vi "PID_controller_18.vi"() -> ()   [LabVIEW 2011]
panel:
  out "Angle (deg)":dbl format="%.1f"
  in  "Local":bool
  in  "Hold":bool
  out "tune_Method":u16(ring) items=["Setpoint", "Angle"]
  in  "Method":u16(ring)=1 items=["Setpoint", "Angle"]
  in  "Setpoint":u16(ring)=2 items=["A", "B", "C", "D"]
  out "do_tune":bool
  in  "Tune":bool
  out "Tune Set Point (torr)":dbl format="%.2f"
  in  "stop":bool
  out "fit":cluster{"element":dbl, "Value":dbl}[](array[cluster])
  out "err_avg":dbl
  out "Setpoint":string
  in  "Ks":dbl
  out "dt(s)":dbl
  out "windup error":dbl
  out "tPrev":dbl
  out "target value":dbl
  out "error(t-t0)":cluster{dbl, "Value":dbl}[](array[cluster])
  out "error":dbl
  out "tStart(s)":dbl
  out "S00":dbl
  out "S10":dbl
  out "S20":dbl
  out "S11":dbl
  out "S01":dbl
  out "weight":dbl[](array[numeric])
  in  "# of points to watch":i32=60
  in  "tSmooth(s)":dbl=4.0
  out "t0":dbl
  out "error(t)":cluster{dbl, "Value":dbl}[](array[cluster])
  out "IO error":errorcluster
  out "first":bool=TRUE
  out "XY Graph":T1(graph)
  out "current value":dbl
  in  "Period (s)":dbl=1.0
  out "dValue":dbl
  out "derivative":dbl
  out "integral":dbl
  in  "Angle (deg)":dbl format="%.1f"
  in  "Kd":dbl=0.4
  in  "Ki":dbl
  in  "Kp":dbl=0.1
  out "P (torr)":dbl format="%.2f"
  in  "Set Point (torr)":dbl format="%.2f"
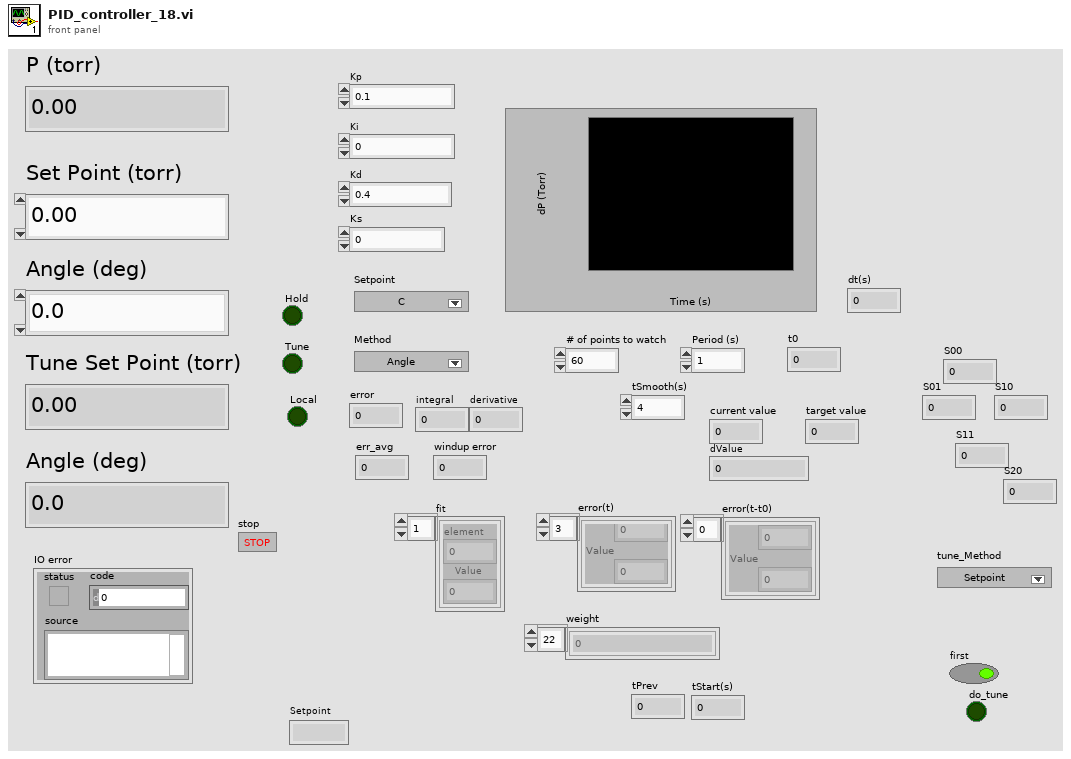
[diagram p1: front panel]
types:
  T1 = cluster{"Value":cluster{"element":dbl, "Value":dbl}[]}[]
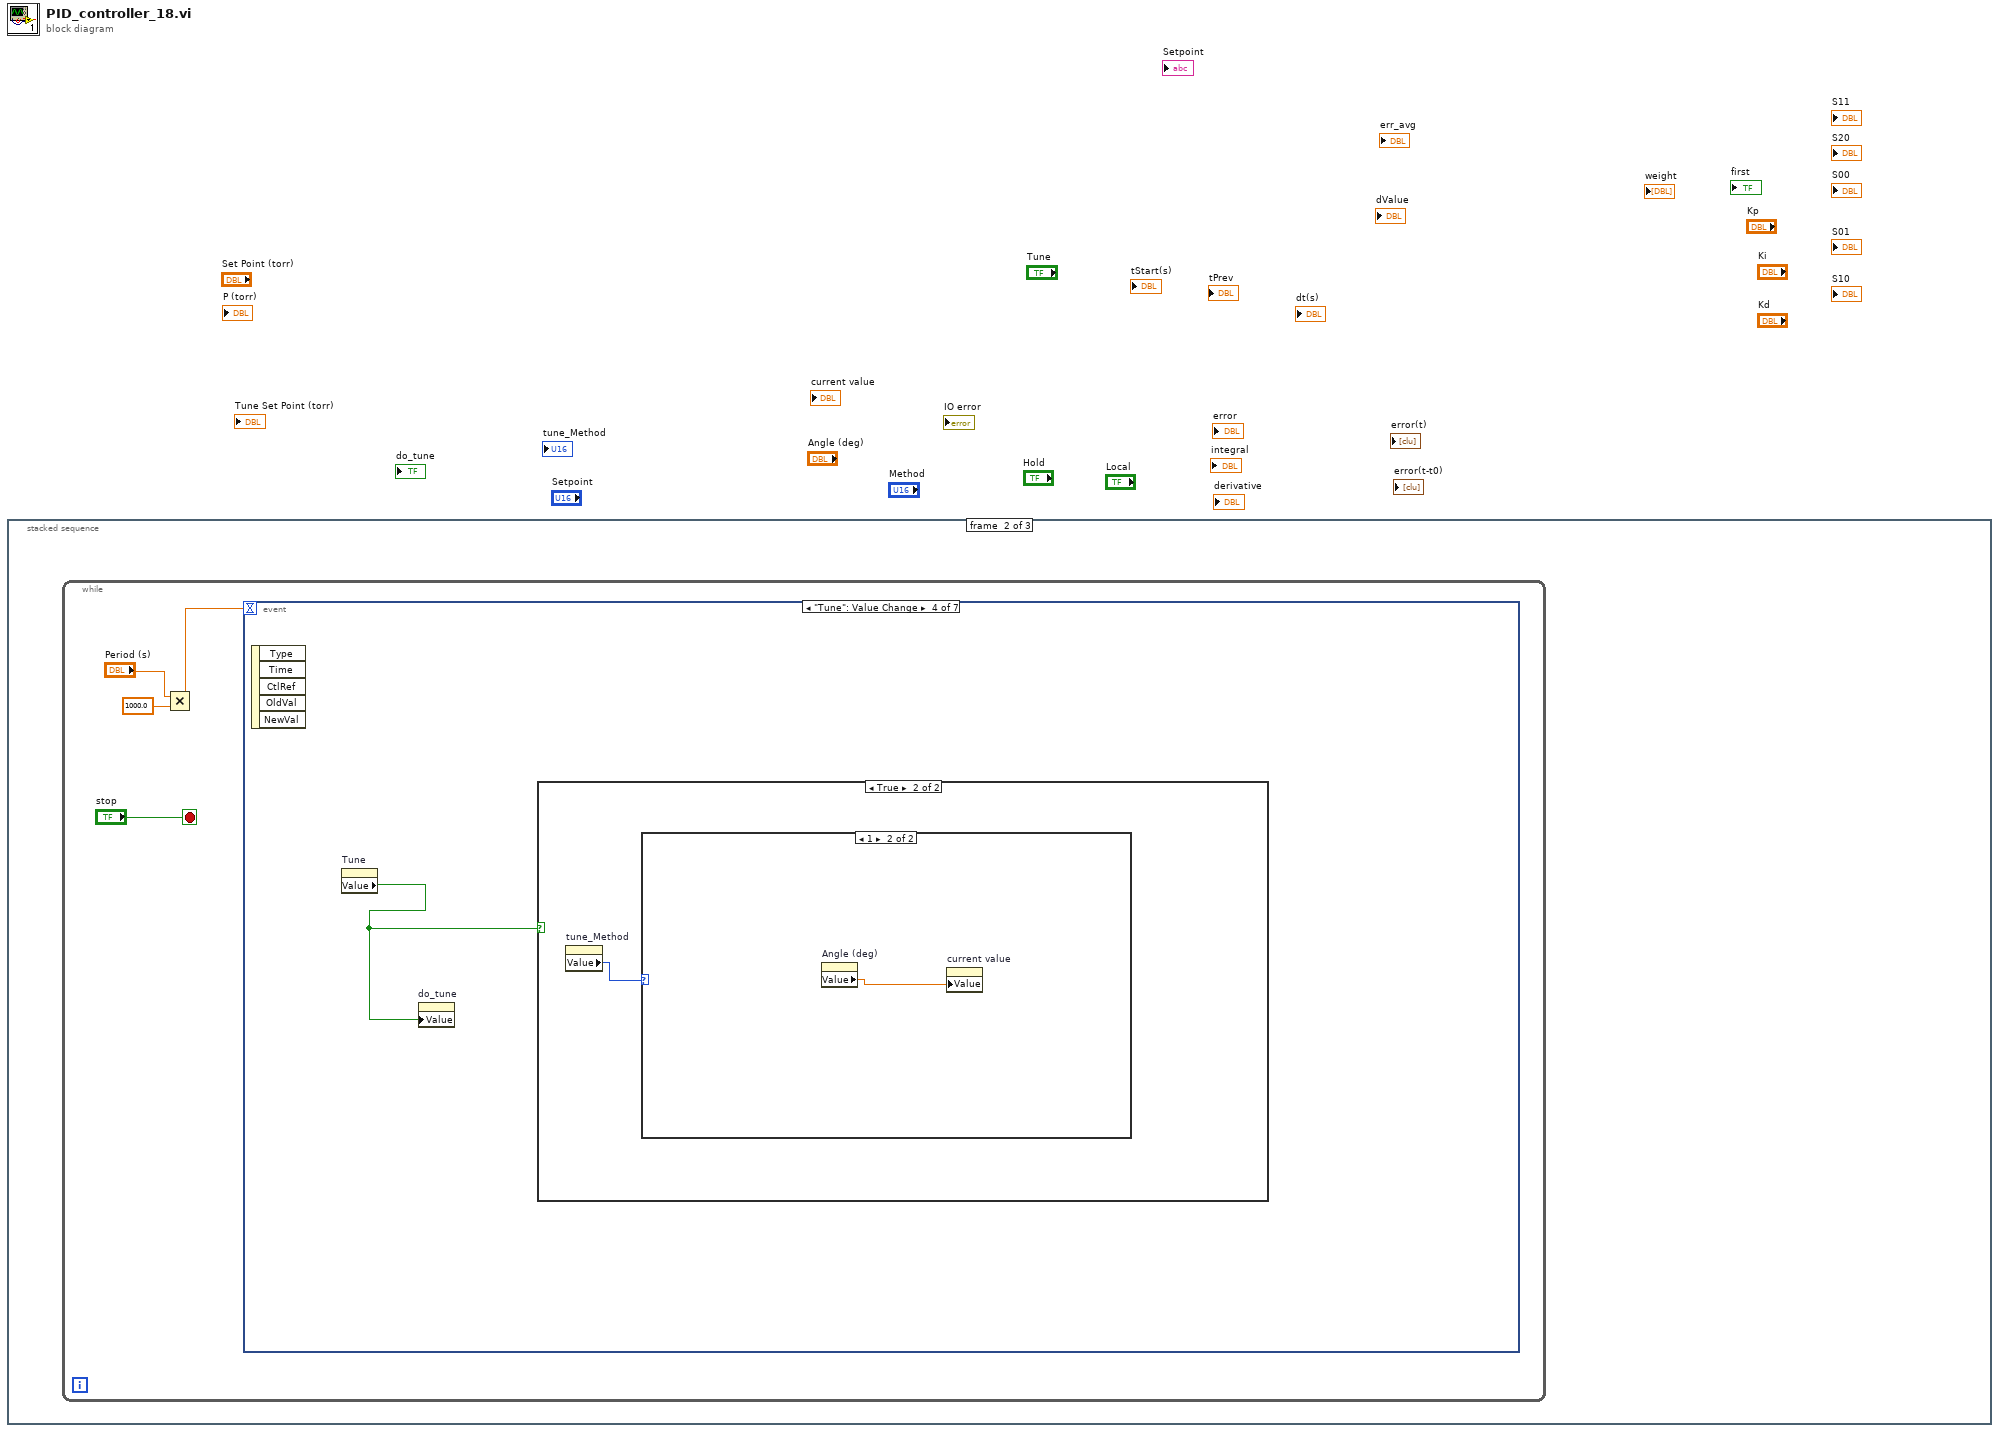
[diagram p0: block diagram]
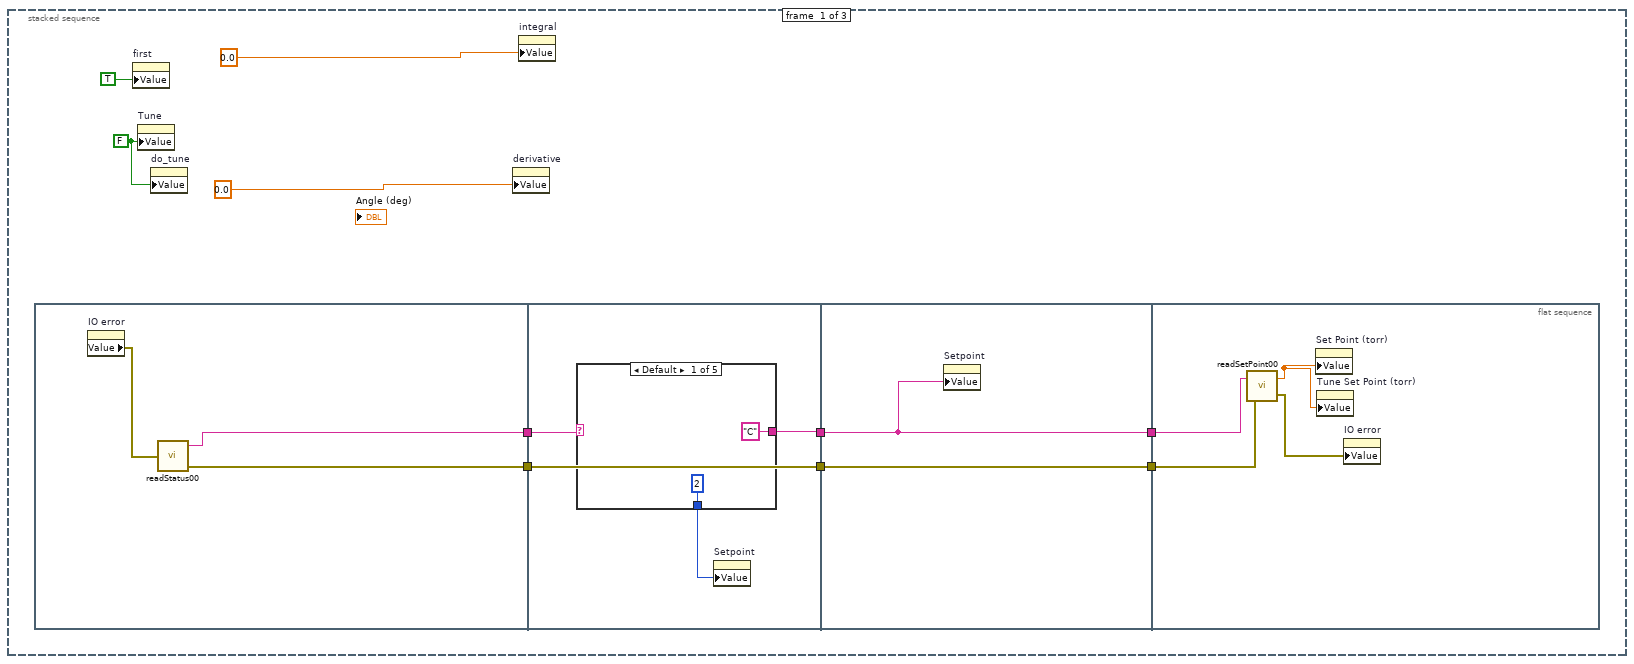
[diagram p2: hidden frame]
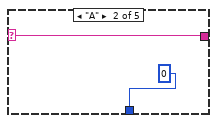
[diagram p3: hidden frame]
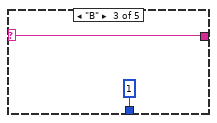
[diagram p4: hidden frame]
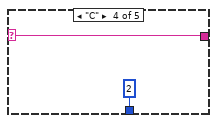
[diagram p5: hidden frame]
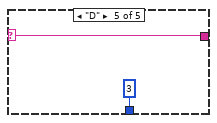
[diagram p6: hidden frame]
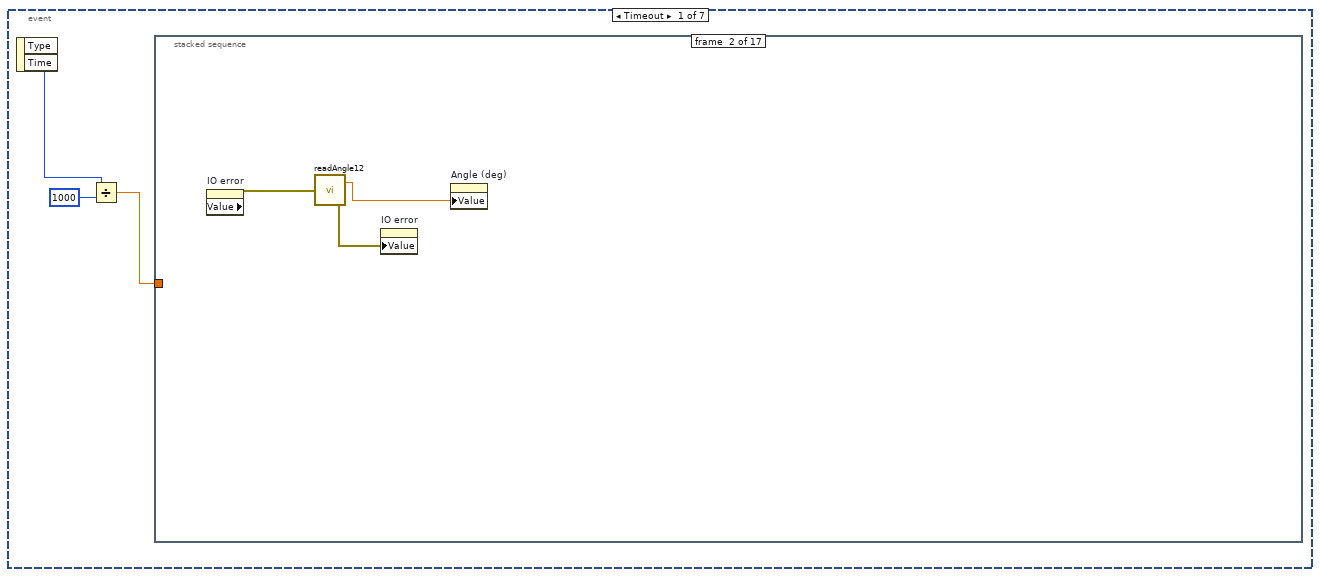
[diagram p7: hidden frame]
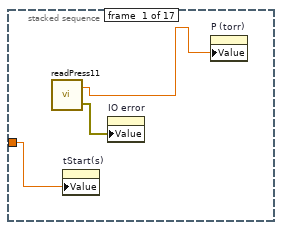
[diagram p8: hidden frame]
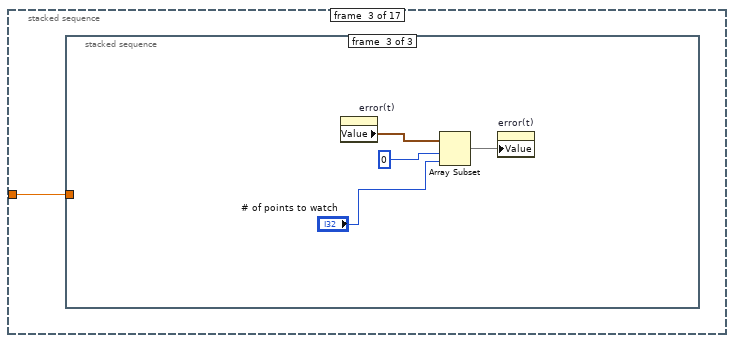
[diagram p9: hidden frame]
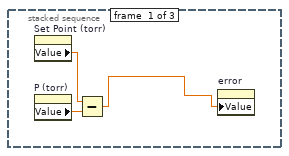
[diagram p10: hidden frame]
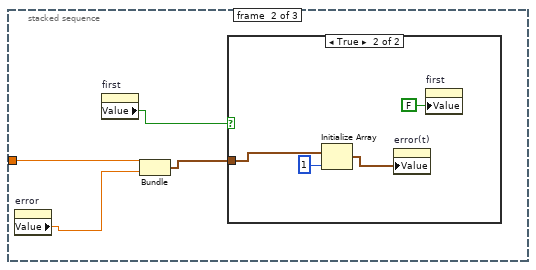
[diagram p11: hidden frame]
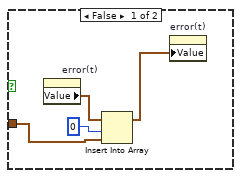
[diagram p12: hidden frame]
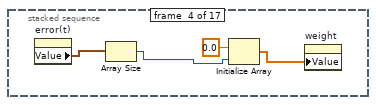
[diagram p13: hidden frame]
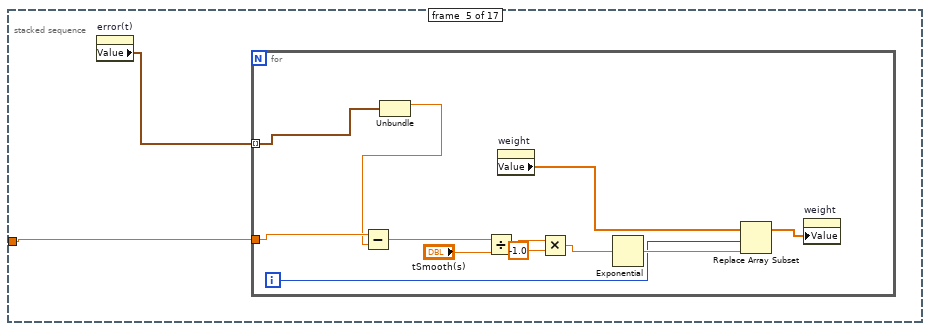
[diagram p14: hidden frame]
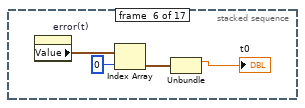
[diagram p15: hidden frame]
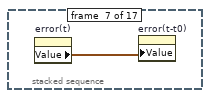
[diagram p16: hidden frame]
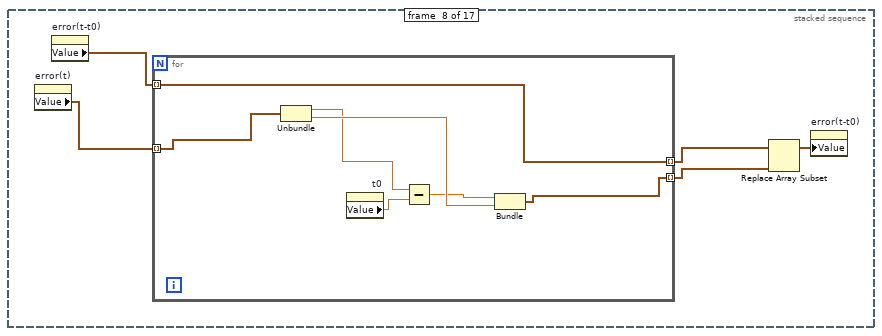
[diagram p17: hidden frame]
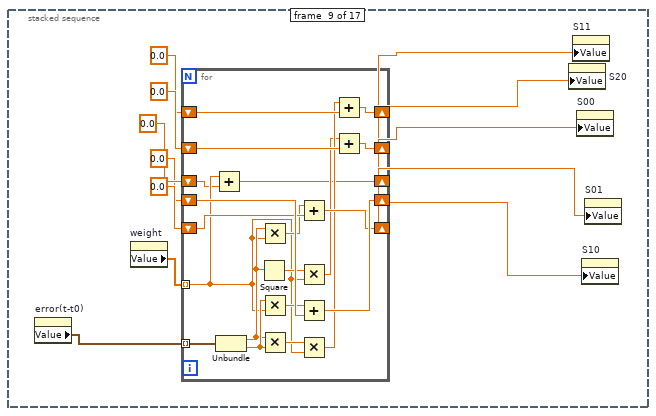
[diagram p18: hidden frame]
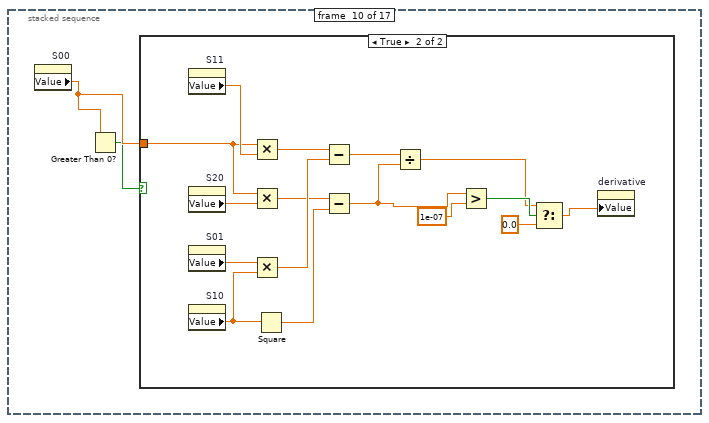
[diagram p19: hidden frame]
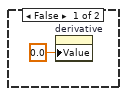
[diagram p20: hidden frame]
diagram:
  n1 = stacked-sequence {
    frame #0 {
      w7 = FALSE ("Tune")
      n2 = flat-sequence {
        tunnel: [w12] -> w6
        tunnel: [w11] -> w5
        tunnel: w6 -> [w16]
        tunnel: [w15] -> w4
        tunnel: w5 -> [w17]
        tunnel: [w17] -> w2
        tunnel: w4 -> [w28]
        tunnel: [w28] -> w3
        tunnel: w2 -> [w29]
        tunnel: [w29] -> w1
        tunnel: w3 -> [w33]
        tunnel: w1 -> [w32]
        frame #0 {
          n3 = property on="IO error" class="Clust (strict)"() -> ("Value"=w13:errorcluster)  [unwired: 2 in, 2 out]
          n4 = call "readStatus00.vi"("error in"=w13) -> ("Setpoint"=w12:string, "error out"=w11:errorcluster)  [unwired: 1 out]
        }
        frame #1 {
          n5 = case shown="Default" w16 {
            selector: w16 -> [_ w21 w22 w24 w26]
            tunnel: ["C" w21 w22 w24 w26] -> w15
            tunnel: [u16 2 ("Ring") u16 0 ("Ring") u16 1 ("Ring") u16 2 ("Ring") u16 3 ("Ring")] -> w14
            frame Default {
            }
            frame "A" {
            }
            frame "B" {
            }
            frame "C" {
            }
            frame "D" {
            }
          }
          n6 = property on="Setpoint" class="Ring (strict)"("Value"=w14) -> ()  [unwired: 2 in, 2 out]
        }
        frame #2 {
          n7 = property on="Setpoint" class="Str"("Value"=w28) -> ()  [unwired: 2 in, 2 out]
        }
        frame #3 {
          n8 = call "readSetPoint00.vi"("error in"=w32, "Setpoint"=w33) -> ("error out"=w31:errorcluster, "P"=w30:dbl)
          n9 = property on="Set Point (torr)" class="DigNum (strict)"("Value"=w30) -> ()  [unwired: 2 in, 2 out]
          n10 = property on="Tune Set Point (torr)" class="DigNum (strict)"("Value"=w30) -> ()  [unwired: 2 in, 2 out]
          n11 = property on="IO error" class="Clust (strict)"("Value"=w31) -> ()  [unwired: 2 in, 2 out]
        }
      }
      n12 = property on="first" class="Bool (strict)"("Value"=TRUE ("first")) -> ()  [unwired: 2 in, 2 out]
      n13 = property on="Tune" class="Bool (strict)"("Value"=w7) -> ()  [unwired: 2 in, 2 out]
      n14 = property on="do_tune" class="Bool (strict)"("Value"=w7) -> ()  [unwired: 2 in, 2 out]
      n15 = property on="derivative" class="DigNum (strict)"("Value"=0.0 ("derivative")) -> ()  [unwired: 2 in, 2 out]
      n16 = property on="integral" class="DigNum (strict)"("Value"=0.0 ("integral")) -> ()  [unwired: 2 in, 2 out]
    }
    frame #1 {
      n17 = while {
        stop <- "stop" stop-if-true
        n18 = Multiply(x="Period (s)", y=1000.0) -> (x*y=w35:dbl)
        n19 = event shown="[3] \"Tune\": Value Change" {
          selector: _ -> [_ _ _ _ _ _ _]
          dyn-events: _ -> [_ _ _ _ _ _ _]
          timeout: w35 -> [_ _ _ _ _ _ _]
          event Timeout {
            n20 = event-data() -> ("Time"=w40:u32)  [unwired: 1 in, 1 out]
            n21 = Divide(x=w40, y=u32 1000) -> (x/y=w38:dbl)
            n22 = stacked-sequence {
              tunnel: w38 -> [w41 _ w47 _ w71 _ _ _ _ _ _ _ _ _ _ _ _]
              frame #0 {
                n23 = call "readPress11.vi"() -> ("P"=w43:dbl, "error out"=w42:errorcluster)  [unwired: 1 in]
                n24 = property on="tStart(s)" class="DigNum (strict)"("Value"=w41) -> ()  [unwired: 2 in, 2 out]
                n25 = property on="IO error" class="Clust (strict)"("Value"=w42) -> ()  [unwired: 2 in, 2 out]
                n26 = property on="P (torr)" class="DigNum (strict)"("Value"=w43) -> ()  [unwired: 2 in, 2 out]
              }
              frame #1 {
                n27 = property on="IO error" class="Clust (strict)"() -> ("Value"=w45:errorcluster)  [unwired: 2 in, 2 out]
                n28 = call "readAngle12.vi"("error in"=w45) -> ("angle"=w46:dbl, "error out"=w44:errorcluster)
                n29 = property on="IO error" class="Clust (strict)"("Value"=w44) -> ()  [unwired: 2 in, 2 out]
                n30 = property on="Angle (deg)" class="DigNum (strict)"("Value"=w46) -> ()  [unwired: 2 in, 2 out]
              }
              frame #2 {
                n31 = stacked-sequence {
                  tunnel: w47 -> [_ w53 _]
                  frame #0 {
                    n32 = property on="Set Point (torr)" class="DigNum (strict)"() -> ("Value"=w49:dbl)  [unwired: 2 in, 2 out]
                    n33 = property on="P (torr)" class="DigNum (strict)"() -> ("Value"=w50:dbl)  [unwired: 2 in, 2 out]
                    n34 = Subtract(x=w49, y=w50) -> (x-y=w48:dbl)
                    n35 = property on="error" class="DigNum (strict)"("Value"=w48) -> ()  [unwired: 2 in, 2 out]
                  }
                  frame #1 {
                    n36 = property on="error" class="DigNum (strict)"() -> ("Value"=w51:dbl)  [unwired: 2 in, 2 out]
                    n37 = property on="first" class="Bool (strict)"() -> ("Value"=w54:bool)  [unwired: 2 in, 2 out]
                    n38 = Bundle(w53, "Value"=w51) -> (w52:cluster{dbl, "Value":dbl})  [unwired: 1 in]
                    n39 = case shown="True" w54 {
                      tunnel: w52 -> [w56 w61]
                      frame False {
                        n40 = property on="error(t)" class="Arr (strict)"() -> ("Value"=w57:cluster{dbl, "Value":dbl}[])  [unwired: 2 in, 2 out]
                        n41 = Insert Into Array(array=w57, index=0, new element=w56) -> (w55:cluster{dbl, "Value":dbl}[])
                        n42 = property on="error(t)" class="Arr (strict)"("Value"=w55) -> ()  [unwired: 2 in, 2 out]
                      }
                      frame True {
                        n43 = Initialize Array(w61, 1 ("dimension size")) -> (w59:cluster{dbl, "Value":dbl}[])
                        n44 = property on="error(t)" class="Arr (strict)"("Value"=w59) -> ()  [unwired: 2 in, 2 out]
                        n45 = property on="first" class="Bool (strict)"("Value"=FALSE ("first")) -> ()  [unwired: 2 in, 2 out]
                      }
                    }
                  }
                  frame #2 {
                    n46 = property on="error(t)" class="Arr (strict)"() -> ("Value"=w64:cluster{dbl, "Value":dbl}[])  [unwired: 2 in, 2 out]
                    n47 = Array Subset(array=w64, index=0, length="# of points to watch") -> (w66:cluster{dbl, "Value":dbl}[])
                    n48 = property on="error(t)" class="Arr (strict)"("Value"=w66) -> ()  [unwired: 2 in, 2 out]
                  }
                }
              }
              frame #3 {
                n49 = property on="error(t)" class="Arr (strict)"() -> ("Value"=w67:cluster{dbl, "Value":dbl}[])  [unwired: 2 in, 2 out]
                n50 = Array Size(array=w67) -> (size(s)=w69:i32)
                n51 = Initialize Array(0.0 ("element"), w69) -> (w70:dbl[])
                n52 = property on="weight" class="Arr (strict)"("Value"=w70) -> ()  [unwired: 2 in, 2 out]
              }
              frame #4 {
                n53 = property on="error(t)" class="Arr (strict)"() -> ("Value"=w72:cluster{dbl, "Value":dbl}[])  [unwired: 2 in, 2 out]
                n54 = for {
                  tunnel: w72 -> [w84] mode=indexing
                  tunnel: w71 -> [w83]
                  i -> [w79]
                  n55 = Unbundle(w84) -> (w82:dbl)  [unwired: 1 out]
                  n56 = Subtract(x=w83, y=w82) -> (x-y=w77:dbl)
                  n57 = Divide(x=w77, y="tSmooth(s)") -> (x/y=w75:dbl)
                  n58 = property on="weight" class="Arr (strict)"() -> ("Value"=w80:dbl[])  [unwired: 2 in, 2 out]
                  n59 = Multiply(x=w75, y=-1.0) -> (x*y=w73:dbl)
                  n60 = Exponential(1:w73) -> (0:w81:dbl)
                  n61 = Replace Array Subset(array=w80, new element=w81, index=w79) -> (w78:dbl[])
                  n62 = property on="weight" class="Arr (strict)"("Value"=w78) -> ()  [unwired: 2 in, 2 out]
                }
              }
              frame #5 {
                n63 = property on="error(t)" class="Arr (strict)"() -> ("Value"=w85:cluster{dbl, "Value":dbl}[])  [unwired: 2 in, 2 out]
                n64 = Index Array(array=w85, index=0) -> (element=w87:cluster{dbl, "Value":dbl})
                n65 = Unbundle(w87) -> (→"t0":dbl)  [unwired: 1 out]
              }
              frame #6 {
                n66 = property on="error(t)" class="Arr (strict)"() -> ("Value"=w89:cluster{dbl, "Value":dbl}[])  [unwired: 2 in, 2 out]
                n67 = property on="error(t-t0)" class="Arr (strict)"("Value"=w89) -> ()  [unwired: 2 in, 2 out]
              }
              frame #7 {
                n68 = property on="error(t)" class="Arr (strict)"() -> ("Value"=w90:cluster{dbl, "Value":dbl}[])  [unwired: 2 in, 2 out]
                n69 = property on="error(t-t0)" class="Arr (strict)"() -> ("Value"=w92:cluster{dbl, "Value":dbl}[])  [unwired: 2 in, 2 out]
                n70 = for {
                  tunnel: w90 -> [w97] mode=indexing
                  tunnel: [w96] -> w91 mode=indexing
                  tunnel: w92 -> [w95] mode=indexing
                  tunnel: [w95] -> w93 mode=indexing
                  n71 = Unbundle(w97) -> (w98:dbl, "Value"=w100:dbl)
                  n72 = property on="t0" class="DigNum (strict)"() -> ("Value"=w101:dbl)  [unwired: 2 in, 2 out]
                  n73 = Subtract(x=w98, y=w101) -> (x-y=w99:dbl)
                  n74 = Bundle(w99, "Value"=w100) -> (w96:cluster{dbl, "Value":dbl})  [unwired: 1 in]
                }
                n75 = Replace Array Subset(array=w93, new element=w91) -> (w94:cluster{dbl, "Value":dbl}[])  [unwired: 1 in]
                n76 = property on="error(t-t0)" class="Arr (strict)"("Value"=w94) -> ()  [unwired: 2 in, 2 out]
              }
              frame #8 {
                n77 = property on="error(t-t0)" class="Arr (strict)"() -> ("Value"=w113:cluster{dbl, "Value":dbl}[])  [unwired: 2 in, 2 out]
                n78 = property on="weight" class="Arr (strict)"() -> ("Value"=w106:dbl[])  [unwired: 2 in, 2 out]
                n79 = for {
                  tunnel: w113 -> [w129] mode=indexing
                  shift-right: [w130] -> w111
                  shift-left: 0.0 -> [w133]
                  shift-right: [w126] -> w108
                  shift-left: 0.0 -> [w132]
                  shift-right: [w125] -> w109
                  shift-left: 0.0 -> [w131]
                  shift-right: [w127] -> w112
                  shift-left: 0.0 -> [w128]
                  tunnel: w106 -> [w116] mode=indexing
                  shift-right: [w114] -> w110
                  shift-left: 0.0 -> [w115]
                  n80 = Add(x=w116, y=w115) -> (x+y=w114:dbl)
                  n81 = Unbundle(w129) -> (w118:dbl, "Value"=w124:dbl)
                  n82 = Square(x=w118) -> (x^2=w120:dbl)
                  n83 = Multiply(x=w118, y=w116) -> (x*y=w117:dbl)
                  n84 = Multiply(x=w124, y=w116) -> (x*y=w123:dbl)
                  n85 = Multiply(x=w118, y=w124) -> (x*y=w122:dbl)
                  n86 = Add(x=w117, y=w128) -> (x+y=w127:dbl)
                  n87 = Multiply(x=w120, y=w116) -> (x*y=w119:dbl)
                  n88 = Add(x=w123, y=w133) -> (x+y=w130:dbl)
                  n89 = Multiply(x=w122, y=w116) -> (x*y=w121:dbl)
                  n90 = Add(x=w121, y=w132) -> (x+y=w126:dbl)
                  n91 = Add(x=w119, y=w131) -> (x+y=w125:dbl)
                }
                n92 = property on="S20" class="DigNum (strict)"("Value"=w109) -> ()  [unwired: 2 in, 2 out]
                n93 = property on="S11" class="DigNum (strict)"("Value"=w108) -> ()  [unwired: 2 in, 2 out]
                n94 = property on="S00" class="DigNum (strict)"("Value"=w110) -> ()  [unwired: 2 in, 2 out]
                n95 = property on="S10" class="DigNum (strict)"("Value"=w112) -> ()  [unwired: 2 in, 2 out]
                n96 = property on="S01" class="DigNum (strict)"("Value"=w111) -> ()  [unwired: 2 in, 2 out]
              }
              frame #9 {
                n97 = property on="S00" class="DigNum (strict)"() -> ("Value"=w135:dbl)  [unwired: 2 in, 2 out]
                n98 = Greater Than 0?(x=w135) -> (x > 0?=w134:bool)
                n99 = case shown="True" w134 {
                  tunnel: w135 -> [_ w144]
                  frame False {
                    n100 = property on="derivative" class="DigNum (strict)"("Value"=0.0 ("derivative")) -> ()  [unwired: 2 in, 2 out]
                  }
                  frame True {
                    n101 = property on="S11" class="DigNum (strict)"() -> ("Value"=w146:dbl)  [unwired: 2 in, 2 out]
                    n102 = property on="S20" class="DigNum (strict)"() -> ("Value"=w145:dbl)  [unwired: 2 in, 2 out]
                    n103 = property on="S01" class="DigNum (strict)"() -> ("Value"=w143:dbl)  [unwired: 2 in, 2 out]
                    n104 = property on="S10" class="DigNum (strict)"() -> ("Value"=w147:dbl)  [unwired: 2 in, 2 out]
                    n105 = Multiply(x=w144, y=w146) -> (x*y=w152:dbl)
                    n106 = Multiply(x=w144, y=w145) -> (x*y=w150:dbl)
                    n107 = Multiply(x=w143, y=w147) -> (x*y=w151:dbl)
                    n108 = Square(x=w147) -> (x^2=w149:dbl)
                    n109 = Subtract(x=w152, y=w151) -> (x-y=w148:dbl)
                    n110 = Subtract(x=w150, y=w149) -> (x-y=w142:dbl)
                    n111 = Divide(x=w148, y=w142) -> (x/y=w138:dbl)
                    n112 = Greater?(x=w142, y=1e-07) -> (0:w140:bool)
                    n113 = Select(t=w138, s=w140, f=0.0) -> (s? t:f=w139:dbl)
                    n114 = property on="derivative" class="DigNum (strict)"("Value"=w139) -> ()  [unwired: 2 in, 2 out]
                  }
                }
              }
              frame #10 {
                n115 = property on="S00" class="DigNum (strict)"() -> ("Value"=w154:dbl)  [unwired: 2 in, 2 out]
                n116 = Greater Than 0?(x=w154) -> (x > 0?=w153:bool)
                n117 = case shown="True" w153 {
                  tunnel: w154 -> [_ w157]
                  frame False {
                    n118 = property on="err_avg" class="DigNum (strict)"("Value"=0.0 ("Pavg")) -> ()  [unwired: 2 in, 2 out]
                  }
                  frame True {
                    n119 = property on="S01" class="DigNum (strict)"() -> ("Value"=w158:dbl)  [unwired: 2 in, 2 out]
                    n120 = property on="S20" class="DigNum (strict)"() -> ("Value"=w161:dbl)  [unwired: 2 in, 2 out]
                    n121 = property on="S11" class="DigNum (strict)"() -> ("Value"=w159:dbl)  [unwired: 2 in, 2 out]
                    n122 = property on="S11" class="DigNum (strict)"() -> ("Value"=w160:dbl)  [unwired: 2 in, 2 out]
                    n123 = Multiply(x=w158, y=w161) -> (x*y=w166:dbl)
                    n124 = Multiply(x=w157, y=w161) -> (x*y=w163:dbl)
                    n125 = Multiply(x=w160, y=w159) -> (x*y=w167:dbl)
                    n126 = Square(x=w160) -> (x^2=w164:dbl)
                    n127 = Subtract(x=w166, y=w167) -> (x-y=w162:dbl)
                    n128 = Subtract(x=w163, y=w164) -> (x-y=w165:dbl)
                    n129 = Divide(x=w162, y=w165) -> (x/y=w156:dbl)
                    n130 = property on="err_avg" class="DigNum (strict)"("Value"=w156) -> ()  [unwired: 2 in, 2 out]
                  }
                }
              }
              frame #11 {
                n131 = property on="error(t-t0)" class="Arr (strict)"() -> ("Value"=w168:cluster{dbl, "Value":dbl}[])  [unwired: 2 in, 2 out]
                n132 = Array Size(array=w168) -> (size(s)=w169:i32)
                n133 = Greater?(x=w169, y=1) -> (0:w171:bool)
                n134 = case shown="True" w171 {
                  frame False {
                  }
                  frame True {
                    n135 = property on="error(t-t0)" class="Arr (strict)"() -> ("Value"=w183:cluster{dbl, "Value":dbl}[])  [unwired: 2 in, 2 out]
                    n136 = Array Size(array=w183) -> (size(s)=w191:i32)
                    n137 = Index Array(array=w183, index=0) -> (element=w189:cluster{dbl, "Value":dbl})
                    n138 = property on="tSmooth(s)" class="DigNum (strict)"() -> ("Value"=w173:dbl)  [unwired: 2 in, 2 out]
                    n139 = Unbundle(w189) -> (w179:dbl)  [unwired: 1 out]
                    n140 = Decrement(x=w191) -> (x-1=w190:i32)
                    n141 = Index Array(array=w183, index=w190) -> (element=w188:cluster{dbl, "Value":dbl})
                    n142 = Multiply(x=w173, y=2.0) -> (x*y=w172:dbl)
                    n143 = Unbundle(w188) -> (w178:dbl)  [unwired: 1 out]
                    n144 = Subtract(x=w179, y=w172) -> (x-y=w176:dbl)
                    n145 = Greater?(x=w178, y=w176) -> (0:w177:bool)
                    n146 = property on="derivative" class="DigNum (strict)"() -> ("Value"=w187:dbl)  [unwired: 2 in, 2 out]
                    n147 = Select(t=w178, s=w177, f=w176) -> (s? t:f=w175:dbl)
                    n148 = property on="error" class="DigNum (strict)"() -> ("Value"=w185:dbl)  [unwired: 2 in, 2 out]
                    n149 = Multiply(x=w175, y=w187) -> (x*y=w186:dbl)
                    n150 = Add(x=w185, y=w186) -> (x+y=w184:dbl)
                    n151 = Bundle(w179, "Value"=w185) -> (w182:cluster{dbl, "Value":dbl})  [unwired: 1 in]
                    n152 = Bundle(w175, w184) -> (w181:cluster{dbl, dbl})  [unwired: 1 in]
                    n153 = Build Array(w182, w181) -> (→"fit":cluster{dbl, "Value":dbl}[])
                  }
                }
              }
              frame #12 {
                n154 = property on="error" class="DigNum (strict)"() -> ("Value"=w195:dbl)  [unwired: 2 in, 2 out]
                n155 = property on="tPrev" class="DigNum (strict)"() -> ("Value"=w194:dbl)  [unwired: 2 in, 2 out]
                n156 = property on="tStart(s)" class="DigNum (strict)"() -> ("Value"=w193:dbl)  [unwired: 2 in, 2 out]
                n157 = Subtract(x=w193, y=w194) -> (x-y=w199:dbl)
                n158 = property on="dt(s)" class="DigNum (strict)"("Value"=w199) -> ()  [unwired: 2 in, 2 out]
                n159 = property on="integral" class="DigNum (strict)"() -> ("Value"=w197:dbl)  [unwired: 2 in, 2 out]
                n160 = Multiply(x=w195, y=w199) -> (x*y=w196:dbl)
                n161 = Add(x=w196, y=w197) -> (x+y=w198:dbl)
                n162 = property on="integral" class="DigNum (strict)"("Value"=w198) -> ()  [unwired: 2 in, 2 out]
              }
              frame #13 {
                n163 = property on="error" class="DigNum (strict)"() -> ("Value"=w212:dbl)  [unwired: 2 in, 2 out]
                n164 = property on="tune_Method" class="Ring (strict)"() -> ("Value"=w202:u16)  [unwired: 2 in, 2 out]
                n165 = property on="Kp" class="DigNum (strict)"() -> ("Value"=w201:dbl)  [unwired: 2 in, 2 out]
                n166 = property on="integral" class="DigNum (strict)"() -> ("Value"=w204:dbl)  [unwired: 2 in, 2 out]
                n167 = property on="derivative" class="DigNum (strict)"() -> ("Value"=w206:dbl)  [unwired: 2 in, 2 out]
                n168 = property on="Ki" class="DigNum (strict)"() -> ("Value"=w203:dbl)  [unwired: 2 in, 2 out]
                n169 = property on="Kd" class="DigNum (strict)"() -> ("Value"=w205:dbl)  [unwired: 2 in, 2 out]
                n170 = case shown="0, Default" w202 {
                  tunnel: w201 -> [w213 w216]
                  tunnel: [w213 w214] -> w200
                  frame 0, Default {
                  }
                  frame 1 {
                    n171 = Multiply(x=w216, y=-1.0) -> (x*y=w214:dbl)
                  }
                }
                n172 = Multiply(x=w205, y=w206) -> (x*y=w209:dbl)
                n173 = Multiply(x=w203, y=w204) -> (x*y=w208:dbl)
                n174 = Multiply(x=w200, y=w212) -> (x*y=w207:dbl)
                n175 = Add(x=w207, y=w208) -> (x+y=w210:dbl)
                n176 = Add(x=w210, y=w209) -> (x+y=w211:dbl)
                n177 = property on="dValue" class="DigNum (strict)"("Value"=w211) -> ()  [unwired: 2 in, 2 out]
              }
              frame #14 {
                n178 = property on="do_tune" class="Bool (strict)"() -> ("Value"=w217:bool)  [unwired: 2 in, 2 out]
                n179 = case shown="True" w217 {
                  frame False {
                  }
                  frame True {
                    w230 = 90.0 ("y")
                    n180 = property on="dValue" class="DigNum (strict)"() -> ("Value"=w235:dbl)  [unwired: 2 in, 2 out]
                    n181 = property on="current value" class="DigNum (strict)"() -> ("Value"=w236:dbl)  [unwired: 2 in, 2 out]
                    n182 = Add(x=w236, y=w235) -> (x+y=w222:dbl)
                    "target value" <- w222
                    n183 = Less Than 0?(x=w222) -> (x < 0?=w234:bool)
                    n184 = Select(t=0.0, s=w234, f=w222) -> (s? t:f=w231:dbl)
                    n185 = property on="IO error" class="Clust (strict)"() -> ("Value"=w220:errorcluster)  [unwired: 2 in, 2 out]
                    n186 = Greater?(x=w231, y=w230) -> (0:w232:bool)
                    n187 = Select(t=w230, s=w232, f=w231) -> (s? t:f=w219:dbl)
                    n188 = Subtract(x=w219, y=w222) -> (x-y=w229:dbl)
                    "windup error" <- w229
                    n189 = property on="dt(s)" class="DigNum (strict)"() -> ("Value"=w228:dbl)  [unwired: 2 in, 2 out]
                    n190 = property on="current value" class="DigNum (strict)"("Value"=w219) -> ()  [unwired: 2 in, 2 out]
                    n191 = property on="tune_Method" class="Ring (strict)"() -> ("Value"=w221:u16)  [unwired: 2 in, 2 out]
                    n192 = Multiply(x=w229, y=w228) -> (x*y=w227:dbl)
                    n193 = property on="integral" class="DigNum (strict)"() -> ("Value"=w224:dbl)  [unwired: 2 in, 2 out]
                    n194 = Multiply(x="Ks", y=w227) -> (x*y=w225:dbl)
                    n195 = case shown="1" w221 {
                      tunnel: w220 -> [w240 w243]
                      tunnel: w219 -> [w239 w242]
                      tunnel: [w237 w241] -> w218
                      frame 0, Default {
                        n196 = property on="Setpoint" class="Str"() -> ("Value"=w238:string)  [unwired: 2 in, 2 out]
                        n197 = property on="Tune Set Point (torr)" class="DigNum (strict)"("Value"=w239) -> ()  [unwired: 2 in, 2 out]
                        n198 = call "writeSetPoint_00.vi"("error in"=w240, "P (Torr)"=w239, "Setpoint"=w238) -> ("error out"=w237:errorcluster)
                      }
                      frame 1 {
                        n199 = call "setAngle_00.vi"("error in (no error)"=w243, "Angle (deg)"=w242) -> ("error out"=w241:errorcluster)
                      }
                    }
                    n200 = Add(x=w225, y=w224) -> (x+y=w223:dbl)
                    n201 = property on="integral" class="DigNum (strict)"("Value"=w223) -> ()  [unwired: 2 in, 2 out]
                    n202 = property on="IO error" class="Clust (strict)"("Value"=w218) -> ()  [unwired: 2 in, 2 out]
                  }
                }
              }
              frame #15 {
                n203 = property on="fit" class="Arr (strict)"() -> ("Value"=w246:cluster{"element":dbl, "Value":dbl}[])  [unwired: 2 in, 2 out]
                n204 = property on="error(t-t0)" class="Arr (strict)"() -> ("Value"=w245:cluster{dbl, "Value":dbl}[])  [unwired: 2 in, 2 out]
                n205 = Build Cluster Array(w245, w246) -> (→"XY Graph":T1)
              }
              frame #16 {
                n206 = property on="tStart(s)" class="DigNum (strict)"() -> ("Value"=w247:dbl)  [unwired: 2 in, 2 out]
                n207 = property on="tPrev" class="DigNum (strict)"("Value"=w247) -> ()  [unwired: 2 in, 2 out]
              }
            }
          }
          event "Hold": Value Change {
            n208 = event-data() -> ()  [unwired: 1 in, 5 out]
            n209 = property on="Hold" class="Bool (strict)"() -> ("Value"=w248:bool)  [unwired: 2 in, 2 out]
            n210 = case shown="False" w248 {
              frame False {
                n211 = property on="Local" class="Bool (strict)"() -> ("Value"=w249:bool)  [unwired: 2 in, 2 out]
                n212 = case shown="False" w249 {
                  frame False {
                    n213 = property on="IO error" class="Clust (strict)"() -> ("Value"=w253:errorcluster)  [unwired: 2 in, 2 out]
                    n214 = property on="Setpoint" class="Str"() -> ("Value"=w250:string)  [unwired: 2 in, 2 out]
                    n215 = call "readSetPoint00.vi"("error in"=w253, "Setpoint"=w250) -> ("error out"=w252:errorcluster, "P"=w251:dbl)
                    n216 = property on="Tune Set Point (torr)" class="DigNum (strict)"("Value"=w251) -> ()  [unwired: 2 in, 2 out]
                    n217 = property on="Set Point (torr)" class="DigNum (strict)"("Value"=w251) -> ()  [unwired: 2 in, 2 out]
                    n218 = property on="IO error" class="Clust (strict)"("Value"=w252) -> ()  [unwired: 2 in, 2 out]
                  }
                  frame True {
                  }
                }
              }
              frame True {
                n219 = property on="IO error" class="Clust (strict)"() -> ("Value"=w257:errorcluster)  [unwired: 2 in, 2 out]
                n220 = property on="Tune" class="Bool (strict)"("Value"=FALSE ("Tune")) -> ()  [unwired: 2 in, 2 out]
                n221 = property on="Local" class="Bool (strict)"("Value"=FALSE ("Local")) -> ()  [unwired: 2 in, 2 out]
                n222 = call "WriteAdaptorr03.vi"("error in (no error)"=w257, "string to write"="H") -> ("error out"=w256:errorcluster)
                n223 = property on="IO error" class="Clust (strict)"("Value"=w256) -> ()  [unwired: 2 in, 2 out]
              }
            }
          }
          event "Local": Value Change {
            n224 = event-data() -> ()  [unwired: 1 in, 5 out]
            n225 = property on="Local" class="Bool (strict)"() -> ("Value"=w259:bool)  [unwired: 2 in, 2 out]
            n226 = case shown="True" w259 {
              frame False {
                n227 = property on="IO error" class="Clust (strict)"() -> ("Value"=w262:errorcluster)  [unwired: 2 in, 2 out]
                n228 = call "WriteAdaptorr03.vi"("error in (no error)"=w262, "string to write"="H") -> ("error out"=w261:errorcluster)
                n229 = property on="Hold" class="Bool (strict)"("Value"=TRUE ("Hold")) -> ()  [unwired: 2 in, 2 out]
                n230 = property on="IO error" class="Clust (strict)"("Value"=w261) -> ()  [unwired: 2 in, 2 out]
              }
              frame True {
                n231 = property on="IO error" class="Clust (strict)"() -> ("Value"=w266:errorcluster)  [unwired: 2 in, 2 out]
                n232 = call "WriteAdaptorr03.vi"("error in (no error)"=w266, "string to write"="D5") -> ("error out"=w267:errorcluster)
                n233 = property on="Hold" class="Bool (strict)"("Value"=FALSE ("Hold")) -> ()  [unwired: 2 in, 2 out]
                n234 = property on="IO error" class="Clust (strict)"("Value"=w267) -> ()  [unwired: 2 in, 2 out]
              }
            }
          }
          event "Tune": Value Change {
            n235 = event-data() -> ()  [unwired: 1 in, 5 out]
            n236 = property on="Tune" class="Bool (strict)"() -> ("Value"=w268:bool)  [unwired: 2 in, 2 out]
            n237 = property on="do_tune" class="Bool (strict)"("Value"=w268) -> ()  [unwired: 2 in, 2 out]
            n238 = case shown="True" w268 {
              frame False {
                n239 = property on="tune_Method" class="Ring (strict)"() -> ("Value"=w269:u16)  [unwired: 2 in, 2 out]
                n240 = case shown="1" w269 {
                  frame 0, Default {
                    n241 = property on="Set Point (torr)" class="DigNum (strict)"() -> ("Value"=w272:dbl)  [unwired: 2 in, 2 out]
                    n242 = property on="Setpoint" class="Str"() -> ("Value"=w273:string)  [unwired: 2 in, 2 out]
                    n243 = property on="IO error" class="Clust (strict)"() -> ("Value"=w271:errorcluster)  [unwired: 2 in, 2 out]
                    n244 = call "writeSetPoint_00.vi"("error in"=w271, "P (Torr)"=w272, "Setpoint"=w273) -> ("error out"=w270:errorcluster)
                    n245 = property on="IO error" class="Clust (strict)"("Value"=w270) -> ()  [unwired: 2 in, 2 out]
                  }
                  frame 1 {
                    n246 = flat-sequence {
                      frame #0 {
                        n247 = call "WriteAdaptorr03.vi"("string to write"="D5") -> ()  [unwired: 1 in, 1 out]
                      }
                      frame #1 {
                        n248 = property on="Setpoint" class="Str"() -> ("Value"=w276:string)  [unwired: 2 in, 2 out]
                        n249 = Concatenate Strings("Press ", w276, " on AdapTorr") -> (w275:string)
                        n250 = One Button Dialog(message=w275) -> ()  [unwired: 1 in, 1 out]
                      }
                    }
                  }
                }
              }
              frame True {
                n251 = property on="tune_Method" class="Ring (strict)"() -> ("Value"=w279:u16)  [unwired: 2 in, 2 out]
                n252 = case shown="1" w279 {
                  frame 0, Default {
                    n253 = property on="IO error" class="Clust (strict)"() -> ("Value"=w282:errorcluster)  [unwired: 2 in, 2 out]
                    n254 = property on="Setpoint" class="Str"() -> ("Value"=w281:string)  [unwired: 2 in, 2 out]
                    n255 = call "readSetPoint00.vi"("error in"=w282, "Setpoint"=w281) -> ("error out"=w283:errorcluster, "P"=w280:dbl)
                    n256 = property on="Tune Set Point (torr)" class="DigNum (strict)"("Value"=w280) -> ()  [unwired: 2 in, 2 out]
                    n257 = property on="Set Point (torr)" class="DigNum (strict)"("Value"=w280) -> ()  [unwired: 2 in, 2 out]
                    n258 = property on="IO error" class="Clust (strict)"("Value"=w283) -> ()  [unwired: 2 in, 2 out]
                    n259 = property on="current value" class="DigNum (strict)"("Value"=w280) -> ()  [unwired: 2 in, 2 out]
                  }
                  frame 1 {
                    n260 = property on="Angle (deg)" class="DigNum (strict)"() -> ("Value"=w284:dbl)  [unwired: 2 in, 2 out]
                    n261 = property on="current value" class="DigNum (strict)"("Value"=w284) -> ()  [unwired: 2 in, 2 out]
                  }
                }
              }
            }
          }
          event "Set Point (torr)": Value Change {
            n262 = event-data() -> ()  [unwired: 1 in, 5 out]
            n263 = property on="Set Point (torr)" class="DigNum (strict)"() -> ("Value"=w287:dbl)  [unwired: 2 in, 2 out]
            n264 = property on="Setpoint" class="Str"() -> ("Value"=w288:string)  [unwired: 2 in, 2 out]
            n265 = property on="IO error" class="Clust (strict)"() -> ("Value"=w286:errorcluster)  [unwired: 2 in, 2 out]
            n266 = call "writeSetPoint_00.vi"("error in"=w286, "P (Torr)"=w287, "Setpoint"=w288) -> ("error out"=w285:errorcluster)
            n267 = property on="IO error" class="Clust (strict)"("Value"=w285) -> ()  [unwired: 2 in, 2 out]
          }
          event "Setpoint": Value Change {
            n268 = event-data() -> ()  [unwired: 1 in, 5 out]
            n269 = property on="Setpoint" class="Ring (strict)"() -> ("Value"=w293:u16)  [unwired: 2 in, 2 out]
            n270 = case shown="3" w293 {
              tunnel: ["A" "B" "C" "D"] -> w289
              frame 0, Default {
              }
              frame 1 {
              }
              frame 2 {
              }
              frame 3 {
              }
            }
            n271 = property on="Setpoint" class="Str"("Value"=w289) -> ()  [unwired: 2 in, 2 out]
            n272 = property on="IO error" class="Clust (strict)"() -> ("Value"=w290:errorcluster)  [unwired: 2 in, 2 out]
            n273 = call "readSetPoint00.vi"("error in"=w290, "Setpoint"=w289) -> ("error out"=w291:errorcluster, "P"=w292:dbl)
            n274 = property on="Set Point (torr)" class="DigNum (strict)"("Value"=w292) -> ()  [unwired: 2 in, 2 out]
            n275 = property on="Tune Set Point (torr)" class="DigNum (strict)"("Value"=w292) -> ()  [unwired: 2 in, 2 out]
            n276 = property on="IO error" class="Clust (strict)"("Value"=w291) -> ()  [unwired: 2 in, 2 out]
          }
          event "Method": Value Change {
            n277 = event-data() -> ()  [unwired: 1 in, 5 out]
            n278 = property on="Method" class="Ring (strict)"() -> ("Value"=w298:u16)  [unwired: 2 in, 2 out]
            n279 = case shown="1" w298 {
              frame 0, Default {
              }
              frame 1 {
                n280 = property on="do_tune" class="Bool (strict)"() -> ("Value"=w299:bool)  [unwired: 2 in, 2 out]
                n281 = case shown="True" w299 {
                  frame False {
                  }
                  frame True {
                    n282 = flat-sequence {
                      frame #0 {
                        n283 = call "WriteAdaptorr03.vi"("string to write"="D5") -> ()  [unwired: 1 in, 1 out]
                      }
                      frame #1 {
                        n284 = property on="Setpoint" class="Str"() -> ("Value"=w302:string)  [unwired: 2 in, 2 out]
                        n285 = Concatenate Strings("Press ", w302, " on AdapTorr") -> (w301:string)
                        n286 = One Button Dialog(message=w301) -> ()  [unwired: 1 in, 1 out]
                      }
                    }
                  }
                }
              }
            }
            n287 = property on="tune_Method" class="Ring (strict)"("Value"=w298) -> ()  [unwired: 2 in, 2 out]
          }
        }
      }
    }
    frame #2 {
      n288 = property on="tune_Method" class="Ring (strict)"() -> ("Value"=w305:u16)  [unwired: 2 in, 2 out]
      n289 = case shown="1" w305 {
        frame 0, Default {
        }
        frame 1 {
          n290 = flat-sequence {
            frame #0 {
              n291 = property on="IO error" class="Clust (strict)"() -> ("Value"=w307:errorcluster)  [unwired: 2 in, 2 out]
              n292 = call "setLocal_And_Hold_00.vi"("error in (no error)"=w307) -> ("error out"=w306:errorcluster)
              n293 = property on="IO error" class="Clust (strict)"("Value"=w306) -> ()  [unwired: 2 in, 2 out]
            }
            frame #1 {
              n294 = property on="Setpoint" class="Str"() -> ("Value"=w309:string)  [unwired: 2 in, 2 out]
              n295 = Concatenate Strings("Press ", w309, " on AdapTorr") -> (w308:string)
              n296 = One Button Dialog(message=w308) -> ()  [unwired: 1 in, 1 out]
            }
          }
        }
      }
    }
  }
